vi "PH_OceanOpticsSpectrometer.contents.vi"   [LabVIEW 2014, in "PH_OceanOpticsSpectrometer.lvlib"]
doc: "This class is forseen to operate an Ocean Optics spectrometer (Typ HR2000+ or HR4000). \n\nThis class is part of the PHELIX device layer."
uses:
  PH_OceanOpticsSpectrometer.lvlib
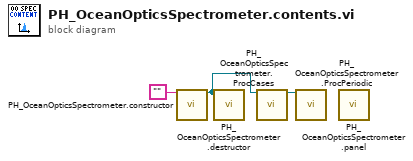
[diagram p0: block diagram]
diagram:
  n1 = call "PH_OceanOpticsSpectrometer.constructor.vi"("name"="") -> ("i ref out"=w1:refnum<vi>)  [unwired: 16 in, 2 out]
  n2 = call "PH_OceanOpticsSpectrometer.destructor.vi"("i ref in"=w1) -> ()  [unwired: 18 in, 1 out]
  n3 = call "PH_OceanOpticsSpectrometer.ProcCases.vi"("i ref in"=w1) -> ("i ref out"=w3:refnum<vi>)  [unwired: 16 in, 2 out]
  n4 = call "PH_OceanOpticsSpectrometer.ProcPeriodic.vi"("i ref in"=w3) -> ()  [unwired: 16 in, 3 out]
  n5 = call "PH_OceanOpticsSpectrometer.panel.vi"() -> ()  [unwired: 19 in, 1 out]
